vi "Square Waves Generator.vi"(1 "Duty Cycle (%)":dbl, 2 "Period (ms)":dbl, 3 "Enable":bool) -> (0 "Signal":bool)   [LabVIEW 2016]
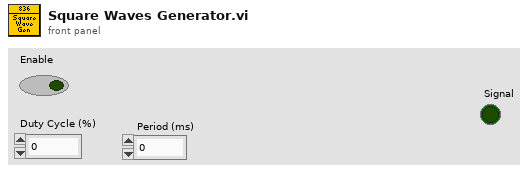
[diagram p1: front panel]
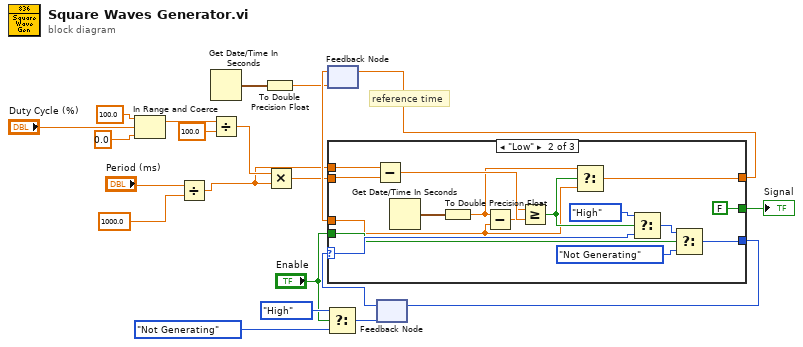
[diagram p0: block diagram]
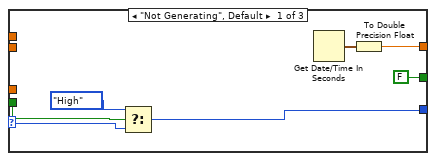
[diagram p2: hidden frame]
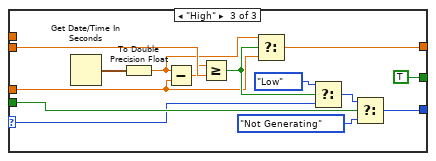
[diagram p3: hidden frame]
diagram:
  # "reference time"
  n1 = In Range and Coerce(upper limit=100.0, x="Duty Cycle (%)", lower limit=0.0) -> (coerced(x)=w10:dbl)  [unwired: 1 out]
  n2 = Divide(x="Period (ms)", y=1000.0) -> (x/y=w2:dbl)
  n3 = Get Date/Time In Seconds() -> (seconds since 1Jan1904=w15:timestamp)
  n4 = Divide(x=w10, y=100.0) -> (x/y=w9:dbl)
  n5 = To Double Precision Float(number=w15) -> (double precision float=w5:dbl)
  n6 = Multiply(x=w9, y=w2) -> (x*y=w8:dbl)
  n7 = Select(t=enum16{"Not Generating", "Low", "High"}."High", s="Enable", f=enum16{"Not Generating", "Low", "High"}."Not Generating") -> (s? t:f=w19:enum16{"Not Generating", "Low", "High"})
  n8 = feedback #1(w5) -> (w16:dbl)
  n9 = feedback #2(w19) -> (w18:enum16{"Not Generating", "Low", "High"})
  n10 = case shown="\"Low\"" w18 {
    selector: w18 -> [w23 w38 w50]
    tunnel: [FALSE FALSE TRUE] -> w17
    tunnel: [w26 w31 w45] -> w4
    tunnel: w16 -> [_ w30 w47]
    tunnel: w2 -> [_ w44 _]
    tunnel: w8 -> [_ w43 w57]
    tunnel: "Enable" -> [w25 w37 w53]
    tunnel: [w22 w34 w49] -> w6
    frame "Not Generating", Default {
      n11 = Select(t=enum16{"Not Generating", "Low", "High"}."High", s=w25, f=w23) -> (s? t:f=w22:enum16{"Not Generating", "Low", "High"})
      n12 = Get Date/Time In Seconds() -> (seconds since 1Jan1904=w27:timestamp)
      n13 = To Double Precision Float(number=w27) -> (double precision float=w26:dbl)
    }
    frame "Low" {
      n14 = Subtract(x=w44, y=w43) -> (x-y=w41:dbl)
      n15 = Get Date/Time In Seconds() -> (seconds since 1Jan1904=w42:timestamp)
      n16 = To Double Precision Float(number=w42) -> (double precision float=w32:dbl)
      n17 = Subtract(x=w32, y=w30) -> (x-y=w40:dbl)
      n18 = Greater Or Equal?(x=w40, y=w41) -> (x >= y?=w33:bool)
      n19 = Select(t=w32, s=w33, f=w30) -> (s? t:f=w31:dbl)
      n20 = Select(t=enum16{"Not Generating", "Low", "High"}."High", s=w33, f=w38) -> (s? t:f=w35:enum16{"Not Generating", "Low", "High"})
      n21 = Select(t=w35, s=w37, f=enum16{"Not Generating", "Low", "High"}."Not Generating") -> (s? t:f=w34:enum16{"Not Generating", "Low", "High"})
    }
    frame "High" {
      n22 = Get Date/Time In Seconds() -> (seconds since 1Jan1904=w56:timestamp)
      n23 = To Double Precision Float(number=w56) -> (double precision float=w46:dbl)
      n24 = Subtract(x=w46, y=w47) -> (x-y=w55:dbl)
      n25 = Greater Or Equal?(x=w55, y=w57) -> (x >= y?=w48:bool)
      n26 = Select(t=w46, s=w48, f=w47) -> (s? t:f=w45:dbl)
      n27 = Select(t=enum16{"Not Generating", "Low", "High"}."Low", s=w48, f=w50) -> (s? t:f=w52:enum16{"Not Generating", "Low", "High"})
      n28 = Select(t=w52, s=w53, f=enum16{"Not Generating", "Low", "High"}."Not Generating") -> (s? t:f=w49:enum16{"Not Generating", "Low", "High"})
    }
  }
  "Signal" <- w17
  n29 = feedback-in #1(w4) -> ()
  n30 = feedback-in #2(w6) -> ()
